vi "SettingsDialog.vi"(8 "error in (no error)":errorcluster, 11 "Settings In":T1) -> (0 "error out":errorcluster, 3 "Settings Out":T1)   [LabVIEW 2018]
uses:
  TypeDef/Settings.ctl
  <vilib>/Utility/miscctls.llb/LVPointTypeDef.ctl
panel:
  in  "Select Printer (double click on printer to select)":i32(listbox)
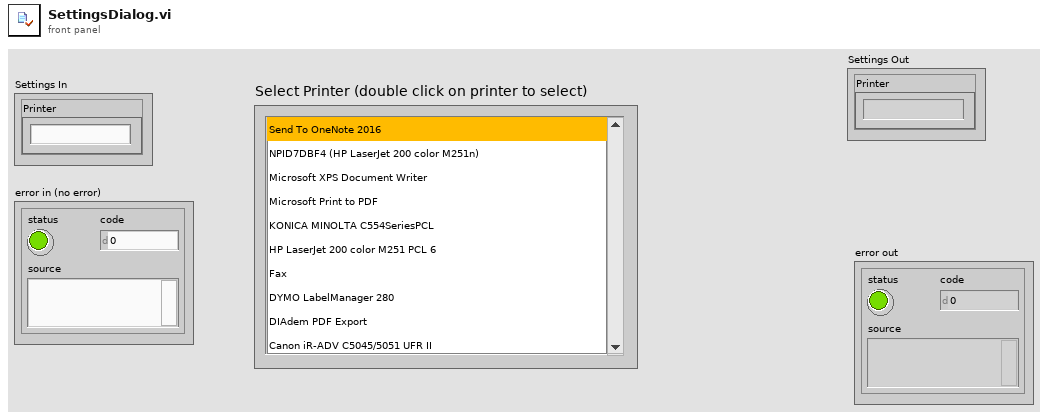
[diagram p1: front panel]
types:
  T1 = typedef "Settings.ctl" = cluster{"Printer":string}
  T2 = typedef "LVPointTypeDef.ctl" = cluster{"Horizontal":i16, "Vertical":i16}
  T3 = cluster{"Printer Name":string, "Default Printer ?":bool}[]
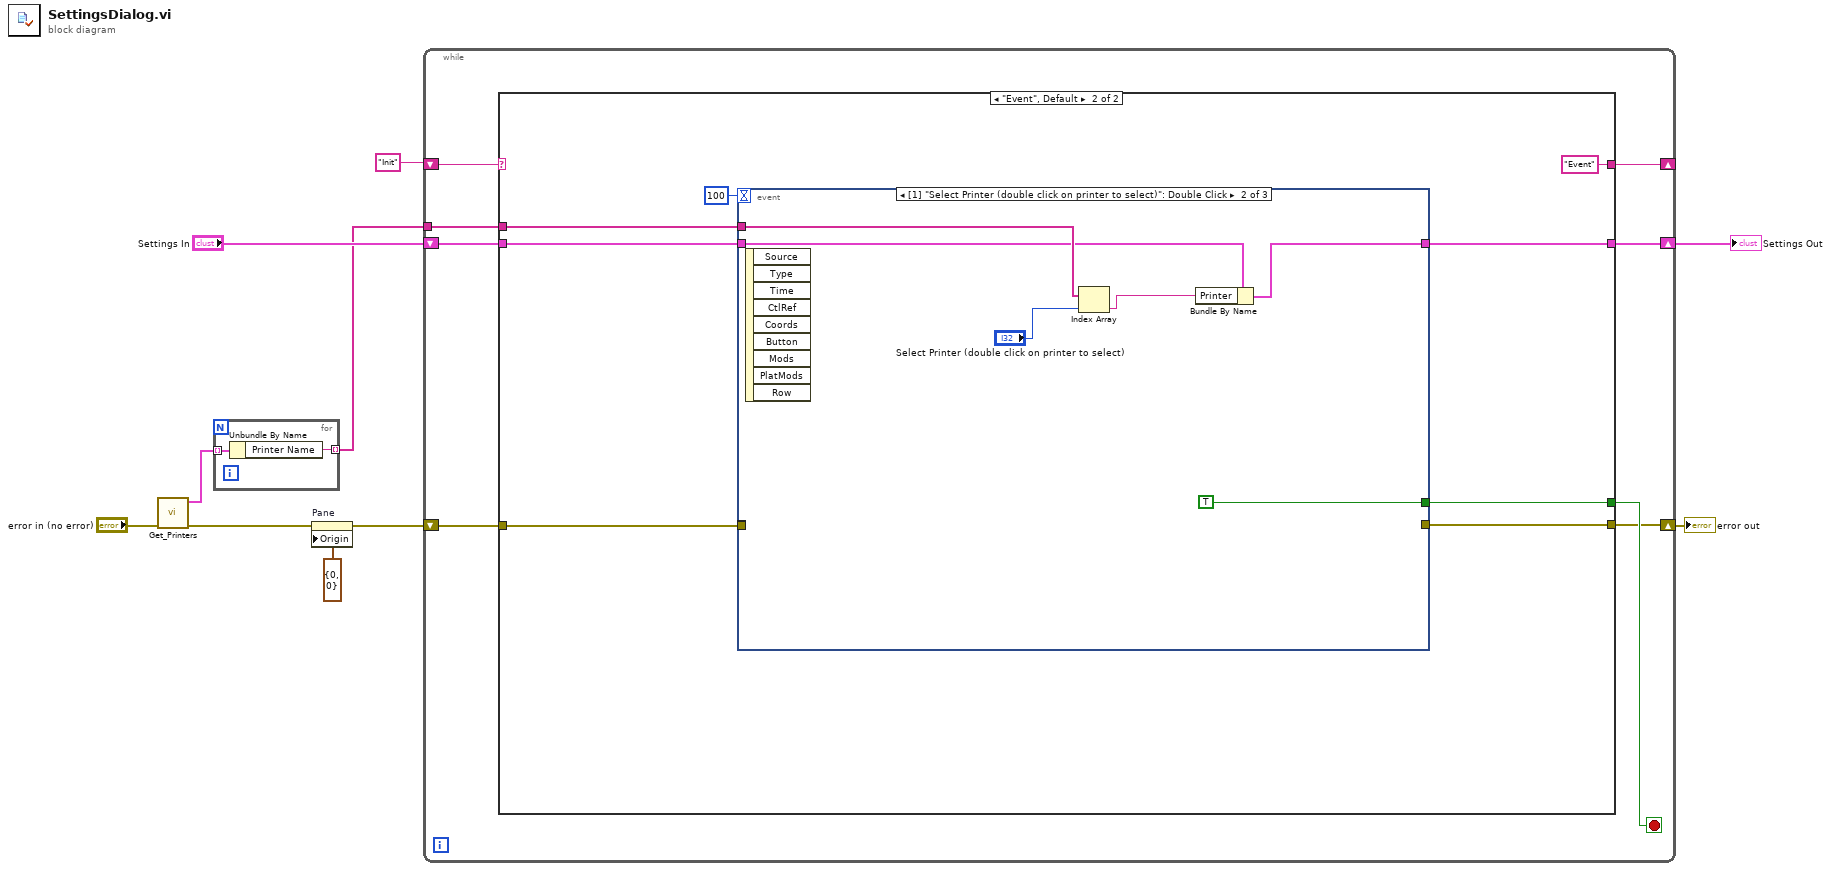
[diagram p0: block diagram]
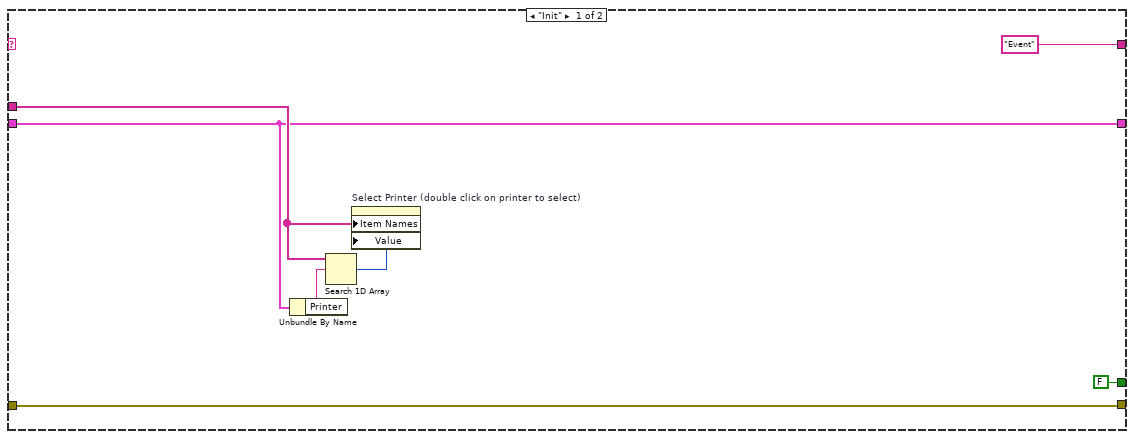
[diagram p2: hidden frame]
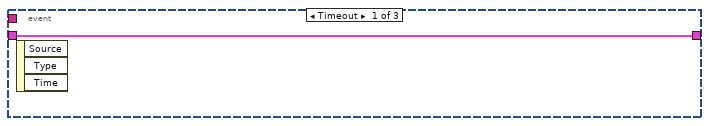
[diagram p3: hidden frame]
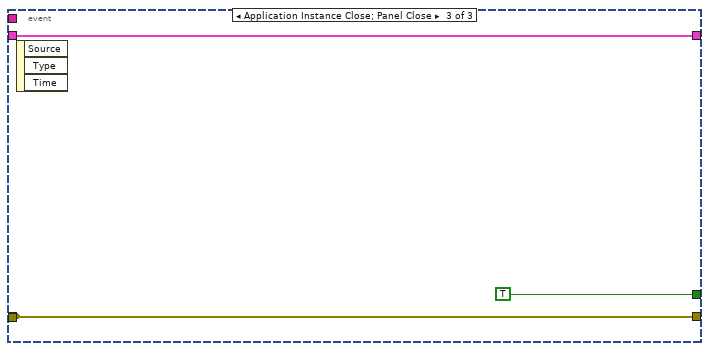
[diagram p4: hidden frame]
diagram:
  n1 = call "Get_Printers.vi"("error in (no error)"="error in (no error)") -> ("error out"=w7:errorcluster, "Printers"=w5:T3)  [unwired: 9 in]
  n2 = for {
    tunnel: w5 -> [w12] mode=indexing
    tunnel: [w11] -> w6 mode=indexing
    n3 = Unbundle By Name(w12) -> ("Printer Name"=w11:string)
  }
  n4 = property on="Pane" class="Pane"(error in=w7, "Origin"=T2 {"Horizontal"=0, "Vertical"=0}) -> (error out=w8:errorcluster)  [unwired: 1 in, 1 out]
  n5 = while {
    shift-right: [w18] -> w1
    shift-left: w8 -> [w19]
    tunnel: w6 -> [w17]
    shift-right: [w13] -> _
    shift-left: "Init" -> [w14]
    shift-right: [w15] -> w4
    shift-left: "Settings In" -> [w16]
    stop <- w20 stop-if-true
    n6 = case shown="\"Event\", Default" w14 {
      tunnel: [FALSE w35] -> w20
      tunnel: w19 -> [w22 w34]
      tunnel: [w22 w33] -> w18
      tunnel: w17 -> [w25 w31]
      tunnel: w16 -> [w23 w30]
      tunnel: [w23 w29] -> w15
      tunnel: ["Event" "Event"] -> w13
      frame "Init" {
        n7 = Unbundle By Name(w23) -> ("Printer"=w27:string)
        n8 = Search 1D Array(1D array=w25, element=w27) -> (index of element=w26:i32)  [unwired: 1 in]
        n9 = property on="Select Printer (double click on printer to select)" class="LstBox (strict)"("Item Names"=w25, "Value"=w26) -> ()  [unwired: 2 in, 2 out]
      }
      frame "Event", Default {
        n10 = event shown="[1] \"Select Printer (double click on printer to select)\": Double Click" {
          selector: _ -> [_ _ _]
          dyn-events: _ -> [_ _ _]
          timeout: 100 -> [_ _ _]
          tunnel: [_ TRUE TRUE] -> w35
          tunnel: w30 -> [w36 w39 w43]
          tunnel: w31 -> [_ w41 _]
          tunnel: [_ _ w45] -> _
          tunnel: w34 -> [_ _ w45]
          tunnel: [_ _ w45] -> w33
          tunnel: [w36 w38 w43] -> w29
          event Timeout {
            n11 = event-data() -> ()  [unwired: 1 in, 3 out]
          }
          event "Select Printer (double click on printer to select)": Double Click {
            n12 = event-data() -> ()  [unwired: 1 in, 9 out]
            n13 = Index Array(array=w41, index="Select Printer (double click on printer to select)") -> (element=w37:string)
            n14 = Bundle By Name(cluster=w39, "Printer"=w37) -> (w38:T1)
          }
          event Application Instance Close; Panel Close {
            n15 = event-data() -> ()  [unwired: 1 in, 3 out]
          }
        }
      }
    }
  }
  "Settings Out" <- w4
  "error out" <- w1
